vi "SALVA BOLLETTINO.vi"(8 "error out":errorcluster, 10 "Array":string[](array[string]), 11 "Refnum in":T1) -> (0 "error out 2":errorcluster, 3 "connection reference":T1)   [LabVIEW 2019]
uses:
  <vilib>/addons/database/Connection.llb/Conn ObjectReference.ctl
  <vilib>/addons/database/Connection.llb/Conn Execute.vi
  <vilib>/addons/database/Recordset.llb/Rec Destroy - Connection.vi
  <vilib>/addons/database/NI_Database_API.lvlib
panel:
  out "size(s) 2":i32
  out "size(s)":i32
  out "String out":string
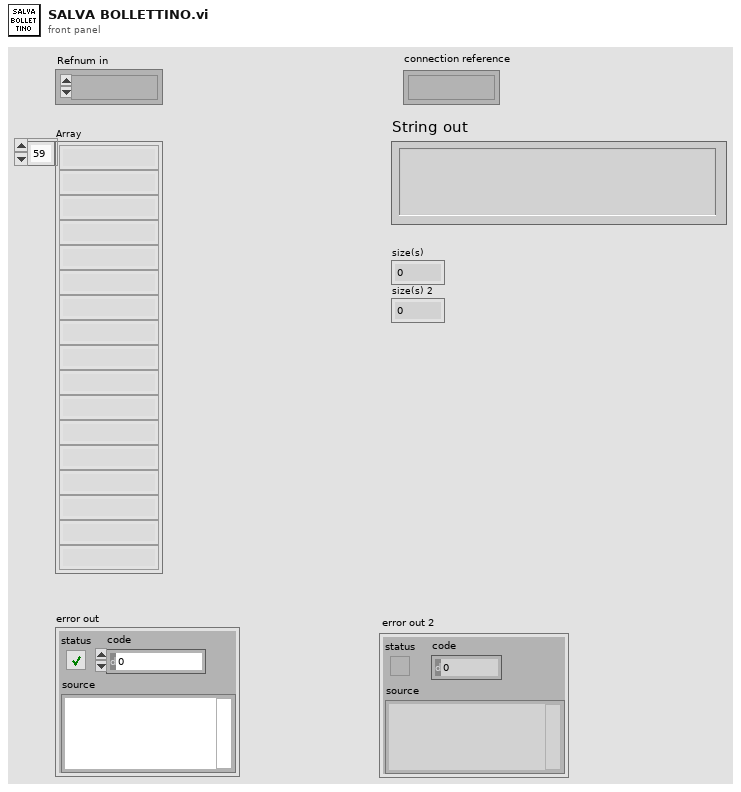
[diagram p1: front panel]
types:
  T1 = typedef "NI_Database_API.lvlib/Conn ObjectReference.ctl" = refnum<k1>
  T2 = typedef "NI_Database_API.lvlib/Rec ObjectReference.ctl" = refnum<k1>
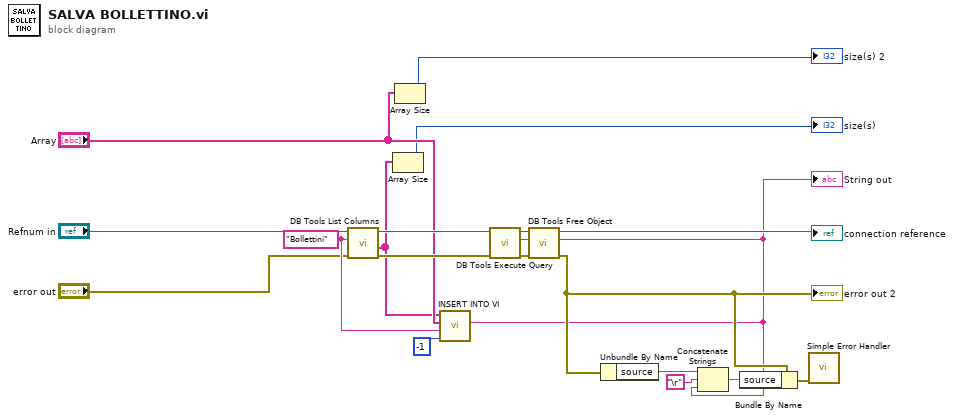
[diagram p0: block diagram]
diagram:
  w19 = "Bollettini" ("table")
  n1 = call <vilib>:"DB Tools List Columns.vi"("error in (no error)"="error out", "table"=w19, "connection reference"="Refnum in") -> ("error out"=w17:errorcluster, "columns"=w10:string[], "connection reference out"=w16:T1)  [unwired: 1 in, 1 out]
  n2 = Array Size(array=w10) -> (size(s)=→"size(s)":i32)
  n3 = Array Size(array="Array") -> (size(s)=→"size(s) 2":i32)
  n4 = call <userlib>:"INSERT INTO VI.vi"("length"=-1, "TABELLA"=w19, "Array"="Array", "columns"=w10) -> ("String out"=w1:string)  [unwired: 7 in]
  "String out" <- w1
  n5 = call-poly <vilib>:"DB Tools Execute Query.vi"("error in (no error)"=w17, "SQL query"=w1, "connection reference"=w16) -> ("error out"=w14:errorcluster, "recordset reference"=w15:T2)  [unwired: 5 in]
  n6 = call-poly <vilib>:"DB Tools Free Object.vi"("error in (no error)"=w14, "recordset reference"=w15) -> ("error out"=w2:errorcluster, "connection reference"=→"connection reference":T1)  [unwired: 8 in]
  "error out 2" <- w2
  n7 = Unbundle By Name(w2) -> ("source"=w6:string)
  n8 = Concatenate Strings(w6, "\r" ("Carriage Return Constant"), w1) -> (w4:string)
  n9 = Bundle By Name(cluster=w2, "source"=w4) -> (w3:errorcluster)
  n10 = call <vilib>:"Simple Error Handler.vi"("error in (no error)"=w3) -> ()  [unwired: 4 in, 5 out]
